vi "Write Data.vi"(8 "error in (no error)":errorcluster, 9 "Publication Time":timestamp, 10 "Value":variant, 11 "TerminalCaptionBinding In":refnum<class "TerminalCaptionBinding.lvclass">) -> (0 "error out":errorcluster, 3 "TerminalCaptionBinding Out":refnum<class "TerminalCaptionBinding.lvclass">)   [LabVIEW 2020, in "TerminalCaptionBinding.lvclass"]
doc: "写入数据"
uses:
  TerminalCaptionBinding.lvclass
  TerminalPropertyBinding/TerminalPropertyBinding.lvclass/TerminalPropertyBinding.ctl
  <vilib>/Utility/error.llb/Error Cluster From Error Code.vi
  <vilib>/ErrorRing/Error Ring.xnode
  TerminalPropertyBinding/TerminalPropertyBinding.lvclass
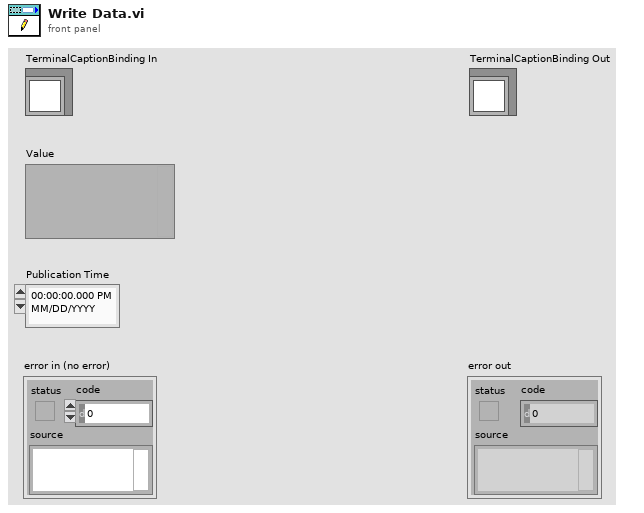
[diagram p1: front panel]
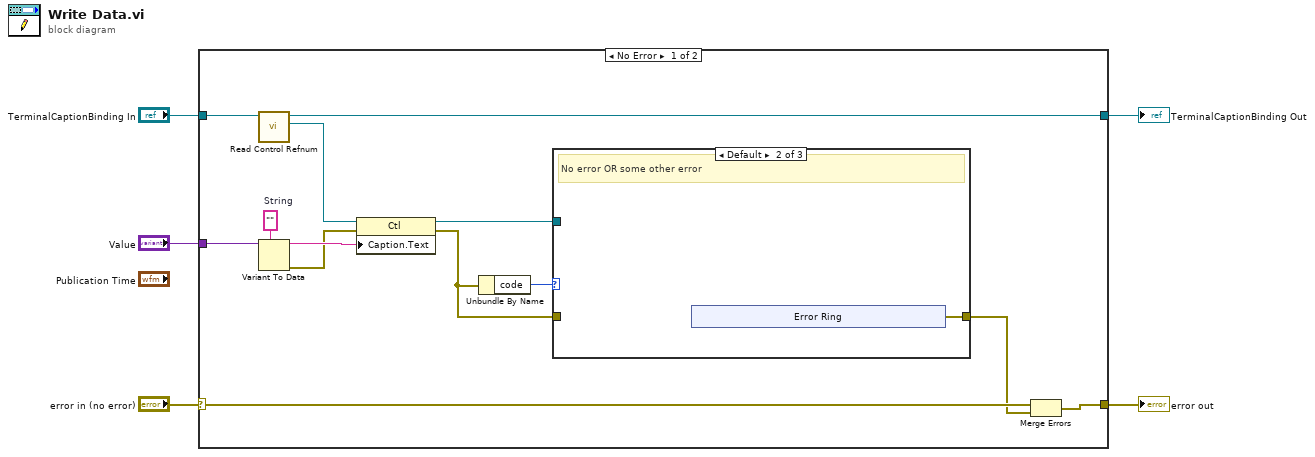
[diagram p0: block diagram]
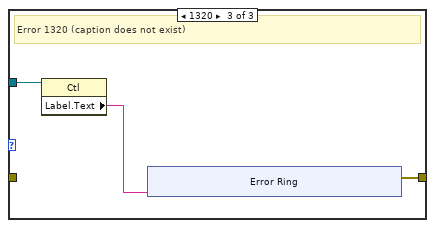
[diagram p3: hidden frame]
diagram:
  n1 = case shown="No Error" "error in (no error)" {
    selector: "error in (no error)" -> [w7 w36]
    tunnel: "TerminalCaptionBinding In" -> [w18 w37]
    tunnel: "Value" -> [w16 _]
    tunnel: [w12 w37] -> w3
    tunnel: [w8 w36] -> w1
    frame No Error {
      w15 = ""  # String
      n2 = call "Read Control Refnum.vi"("TerminalReferenceBinding in"=w18) -> ("Ctl Refnum"=w11:refnum<vi>, "TerminalReferenceBinding out"=w12:refnum<class "TerminalCaptionBinding.lvclass">)  [unwired: 9 in]
      n3 = Variant To Data(type=w15, Variant=w16) -> (data=w17:string, error out=w14:errorcluster)  [unwired: 1 in]
      n4 = property class="Ctl"(reference=w11, error in=w14, "Caption.Text"=w17) -> (reference out=w13:refnum<vi>, error out=w10:errorcluster)
      n5 = Unbundle By Name(w10) -> ("code"=w9:i32)
      n6 = case shown="Default" w9 {
        tunnel: [w19 w20 w28] -> w6
        tunnel: w13 -> [_ _ w27]
        tunnel: w10 -> [w19 _ _]
        frame 0 {
          # "No error"
        }
        frame Default {
          # "No error OR some other error"
          n7 = xnode "Error Ring"() -> ("error out"=w20:errorcluster)
        }
        frame 1320 {
          # "Error 1320 (caption does not exist)"
          n8 = property class="Ctl"(reference=w27) -> ("Label.Text"=w26:string)  [unwired: 1 in, 2 out]
          n9 = xnode "Error Ring"("parameter 0"=w26) -> ("error out"=w28:errorcluster)
        }
      }
      n10 = Merge Errors(w7, w6) -> (w8:errorcluster)
    }
    frame Error {
    }
  }
  "error out" <- w1
  "TerminalCaptionBinding Out" <- w3
